vi "Flush all Infinite Messages.vi"(8 "error in (no error)":errorcluster, 11 "Guardian in":refnum<class "Guardian.lvclass">) -> (0 "error out":errorcluster, 3 "Guardian out":refnum<class "Guardian.lvclass">)   [LabVIEW 2026]
uses:
  Guardian.lvclass
  Ancestor/Ancestor/Infinite Message Selector.ctl
  Ancestor/Ancestor/Ancestor.lvclass
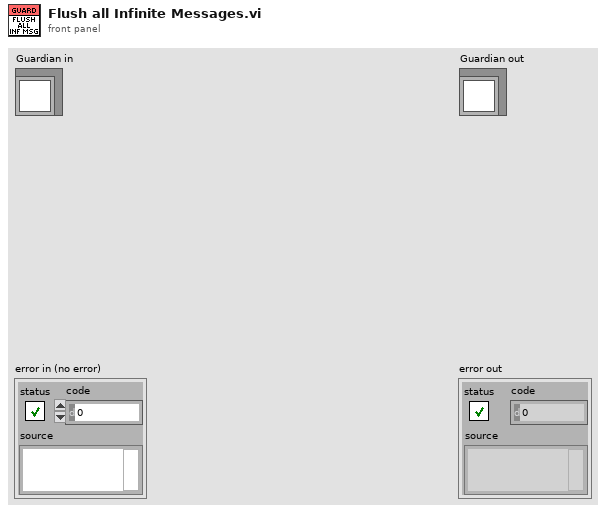
[diagram p1: front panel]
types:
  T1 = typedef "TALOS.lvlib/Ancestor.lvlib/Ancestor.lvclass/Infinite Message Selector.ctl" = enum16{"Start", "Stop", "Check", "Flush (Stop all)", "Init"}
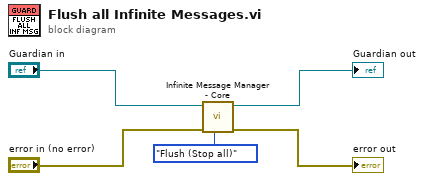
[diagram p0: block diagram]
diagram:
  n1 = call-dynamic "Infinite Message Manager - Core.vi"("Infinite Message Selector"=Infinite_Message_Selector."Flush (Stop all)", "error in (no error)"="error in (no error)", "Ancestor in"="Guardian in") -> ("error out"=→"error out":errorcluster, "Ancestor out"=→"Guardian out":refnum<class "Guardian.lvclass">)  [unwired: 6 in, 1 out]
